vi "test_CCD_Teardown_Testenvironment.vi"(8 "error in":errorcluster, 11 "CCD in":refnum<class "CCD.lvclass">) -> (0 "error out":errorcluster, 2 "device is open?":bool)   [LabVIEW 2023]
uses:
  Source/Libraries/DeviceManager/DeviceManager.lvlib
  Source/Classes/CCD/CCD.lvclass
panel:
  # "Connector Pane"
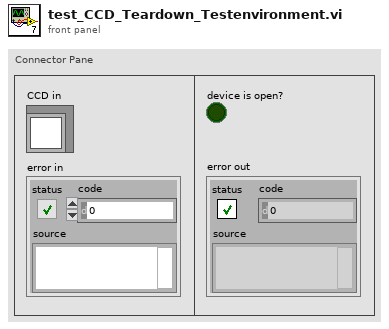
[diagram p1: front panel]
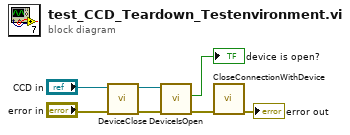
[diagram p0: block diagram]
diagram:
  n1 = call-dynamic "DeviceClose.vi"("error in (no error)"="error in", "CCD in"="CCD in") -> ("error out"=w4:errorcluster, "CCD out"=w5:refnum<class "CCD.lvclass">)  [unwired: 6 in, 2 out]
  n2 = call-dynamic "DeviceIsOpen.vi"("error in (no error)"=w4, "CCD in"=w5) -> ("error out"=w3:errorcluster, "device is open?"=→"device is open?":bool)  [unwired: 6 in, 2 out]
  n3 = call "CloseConnectionWithDevice.vi"("error in (no error)"=w3) -> ("error out"=→"error out":errorcluster)  [unwired: 10 in]
